vi "Registry Logging.vi"() -> ()   [LabVIEW 2018]
uses:
  src/api/Log Levels.ctl
  src/api/GLog.lvlib
  ff44e4a9-c346-414c-ae2a-efcf3ff82913.vi
  c9322c4e-9f12-43bd-adb9-b3674d2f7074.vi
  cbe71786-2e87-4bc7-85be-dae61289713f.vi
  593378fc-b3d1-4ba2-990a-aac09aa27d13.vi
  src/api/configuration/scopes/basic_scope/Basic.lvclass
  src/api/configuration/filters/regex_filter/Regex.lvclass
  src/api/configuration/handlers/file_handler/File Handler.lvclass
  src/api/configuration/formatters/format_string_formatter/Format String.lvclass
  src/api/configuration/filters/regex_filter/New (Element).vi
  src/api/configuration/scopes/basic_scope/New (Element).vi
panel:
  out "ms timer":u32[](array[numeric])
  out "elapsed time":u32[](array[numeric])
  out "iterations":i32[](array[numeric])
  in  "error in (no error)":errorcluster
  out "error out":errorcluster
  in  "total iterations":i32=30
  # "Locals"
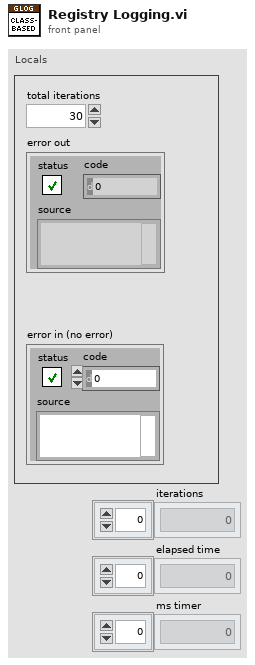
[diagram p1: front panel]
types:
  T1 = typedef "GLog.lvlib/Log Levels.ctl" = enum16{"Trace", "Debug", "Info", "Warning", "Error", "Critical"}
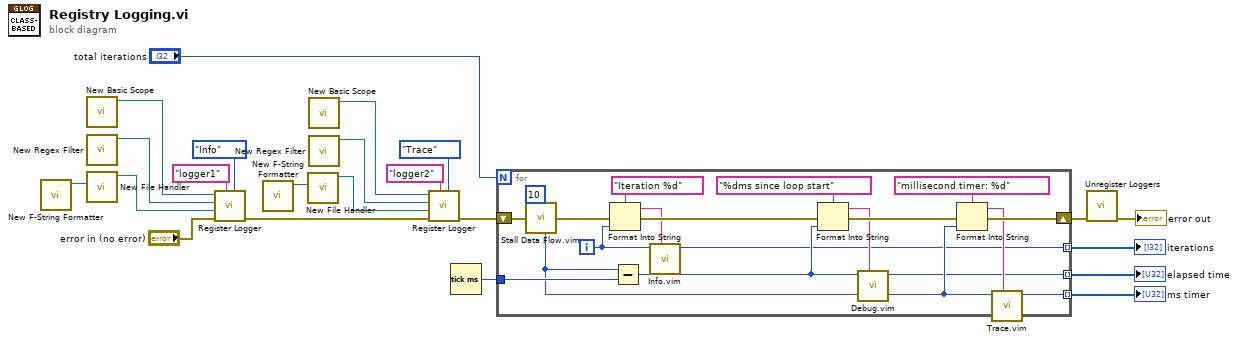
[diagram p0: block diagram]
diagram:
  n1 = call "New F-String Formatter.vi"() -> ("new f-string formatter"=w10:refnum<class "Format String.lvclass">)  [unwired: 11 in]
  n2 = call-poly "New Basic Scope.vi"() -> ("basic scope"=w13:refnum<class "Basic.lvclass">)  [unwired: 11 in]
  n3 = call-poly "New Regex Filter.vi"() -> ("regex out"=w12:refnum<class "Regex.lvclass">)  [unwired: 10 in, 1 out]
  n4 = call "New File Handler.vi"("formatter (JSON)"=w10) -> ("file handler"=w11:refnum<class "File Handler.lvclass">)  [unwired: 10 in]
  n5 = call "Register Logger.vi"("minimum log level (Info)"=Log_Levels."Info" ("minimum log level"), "name (\"Default\")"="logger1" ("name (\"Default\")"), "error in (no error)"="error in (no error)", "log handler (file handler)"=w11, "log filter (none)"=w12, "logger scope (all)"=w13) -> ("error out"=w1:errorcluster)  [unwired: 5 in]
  n6 = call "New F-String Formatter.vi"() -> ("new f-string formatter"=w5:refnum<class "Format String.lvclass">)  [unwired: 11 in]
  n7 = call "New File Handler.vi"("formatter (JSON)"=w5) -> ("file handler"=w6:refnum<class "File Handler.lvclass">)  [unwired: 10 in]
  n8 = call-poly "New Basic Scope.vi"() -> ("basic scope"=w8:refnum<class "Basic.lvclass">)  [unwired: 11 in]
  n9 = call-poly "New Regex Filter.vi"() -> ("regex out"=w7:refnum<class "Regex.lvclass">)  [unwired: 10 in, 1 out]
  n10 = call "Register Logger.vi"("minimum log level (Info)"=Log_Levels."Trace" ("minimum log level"), "name (\"Default\")"="logger2" ("name (\"Default\")"), "error in (no error)"=w1, "log handler (file handler)"=w6, "log filter (none)"=w7, "logger scope (all)"=w8) -> ("error out"=w2:errorcluster)  [unwired: 5 in]
  n11 = Tick Count (ms)() -> (millisecond timer value=w22:u32)
  n12 = for {
    N: "total iterations" -> [_]
    tunnel: w22 -> [w41]
    shift-right: [w34] -> w20
    shift-left: w2 -> [w27]
    tunnel: [w25] -> w18 mode=indexing
    tunnel: [w24] -> w17 mode=indexing
    tunnel: [w23] -> w16 mode=indexing
    i -> [w33]
    n13 = call "Stall Data Flow.vim"("value in"=w27, "milliseconds to wait"=u32 10 ("loop iteration delay [ms]")) -> ("millisecond timer value"=w29:u32, "value out"=w26:errorcluster)
    n14 = Format Into String(format string="Iteration %d" ("message"), error in=w26, w33) -> (resulting string=w32:string, error out=w36:errorcluster)  [unwired: 1 in]
    n15 = Subtract(x=w29, y=w41) -> (x-y=w30:u32)
    n16 = call "Info.vim"("data in (null)"=w33, "message"=w32) -> ("data out"=w25:i32)  [unwired: 9 in]
    n17 = Format Into String(format string="%dms since loop start" ("message"), error in=w36, w30) -> (resulting string=w31:string, error out=w35:errorcluster)  [unwired: 1 in]
    n18 = call "Debug.vim"("data in (null)"=w30, "message"=w31) -> ("data out"=w24:u32)  [unwired: 9 in]
    n19 = Format Into String(format string="millisecond timer: %d" ("message"), error in=w35, w29) -> (resulting string=w28:string, error out=w34:errorcluster)  [unwired: 1 in]
    n20 = call "Trace.vim"("data in (null)"=w29, "message"=w28) -> ("data out"=w23:u32)  [unwired: 9 in]
  }
  "iterations" <- w18
  "elapsed time" <- w17
  "ms timer" <- w16
  n21 = call "Unregister Loggers.vi"("error in (no error)"=w20) -> ("error out"=→"error out":errorcluster)  [unwired: 9 in, 1 out]
